vi "CreateQueueNames.vi"(0 "ModuleAdmin":refnum<class "ModuleAdmin.lvclass">, 5 "QueueNames":string[](array[string])=["QMH", "Class", "SP"], 11 "error in (no error)":errorcluster) -> (4 "ModuleAdmin Out":refnum<class "ModuleAdmin.lvclass">, 6 "QMH Queue Name":string, 8 "Class Queue Name":string, 10 "SP Loop Queue Name":string, 15 "error out":errorcluster)   [LabVIEW 2018, in "MyPlugins.lvlib"]
doc: "This creates or recreates the queue name and obtains a reference to the queue."
uses:
  MyPlugins.lvlib
  <userlib>/NIST/ModuleAdminLib/ModuleAdmin/ModuleAdmin.lvclass
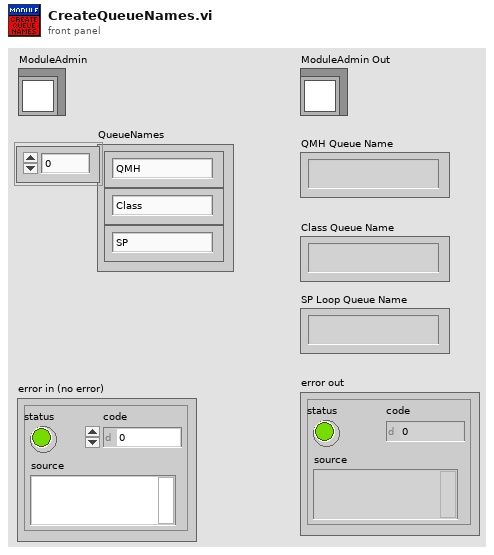
[diagram p1: front panel]
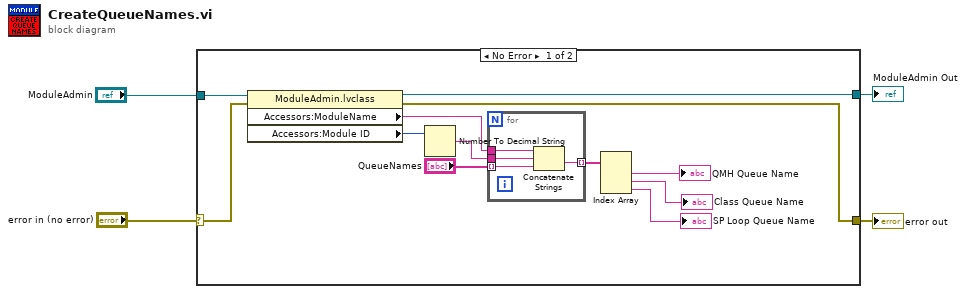
[diagram p0: block diagram]
diagram:
  n1 = case shown="No Error" "error in (no error)" {
    selector: "error in (no error)" -> [w11 w22]
    tunnel: [w10 w22] -> w1
    tunnel: "ModuleAdmin" -> [w6 w21]
    tunnel: [w5 w21] -> w2
    frame No Error {
      n2 = property class="ModuleAdmin.lvclass"(reference=w6, error in=w11) -> (reference out=w5:refnum<class "ModuleAdmin.lvclass">, error out=w10:errorcluster, "Accessors:ModuleName"=w7:string, "Accessors:Module ID"=w8:i32)
      n3 = Number To Decimal String(number=w8) -> (decimal integer string=w9:string)  [unwired: 1 in]
      n4 = for {
        tunnel: [w20] -> w16 mode=indexing
        tunnel: w9 -> [w19]
        tunnel: "QueueNames" -> [w18] mode=indexing
        tunnel: w7 -> [w17]
        n5 = Concatenate Strings(w17, w19, w18) -> (w20:string)
      }
      n6 = Index Array(array=w16) -> (element #1=→"QMH Queue Name":string, element #2=→"Class Queue Name":string, element #3=→"SP Loop Queue Name":string)  [unwired: 3 in]
    }
    frame Error {
    }
  }
  "error out" <- w1
  "ModuleAdmin Out" <- w2
